vi "Read Register.vi"() -> ()   [LabVIEW 2013]
uses:
  HSDIO/MIPI_RFFE/Ctrls/Configuration.ctl
  HSDIO/MIPI_RFFE/Ctrls/ClockDataChannels.ctl
  HSDIO/MIPI_RFFE/Ctrls/RegReadWrite.ctl
  <vilib>/NI_TestStand_SemiconductorModule/NI_TestStand_Semiconductor_Module.lvlibp/PinMap/General/SemiconductorModuleContext.ctl
  <vilib>/NI_TestStand_SemiconductorModule/NI_TestStand_Semiconductor_Module.lvlibp/PinMap/HSDIO/PinsToNIHSDIOSession.vi
  <instrlib>/niHSDIO/niHSDIO.llb/niHSDIO Write Named Waveform (WDT).vi
  <instrlib>/niHSDIO/niHSDIO.llb/niHSDIO Fetch Waveform (WDT).vi
  <vilib>/NI_TestStand_SemiconductorModule/NI_TestStand_Semiconductor_Module.lvlibp
panel:
  in  "Semiconductor Module Context":T1
  in  "Pins":string[](array[string])=["CLK", "SDA", "SETID"]
  out "Converted Data":T2 {"Register" max=31 format="%.0x"; "Slave Address" max=15 format="%.0x"}
  in  "Readback Speed":enum16{"Full Speed", "Half Speed"}(ring)
  in  "Data":T3 {"Register" max=31 format="%.0x"; "Slave Address" max=15 format="%.0x"}
  in  "Configuratation":T4={"Samples to Allocate"=10000, "Oversample Factor"=1, "Clock Channel"=enum."0", "Data Channel"=enum."1"} {"Oversample Factor" min=1 max=254; "Samples to Allocate" min=1}
  out "Waveform Graph":digitalwaveform(graph)
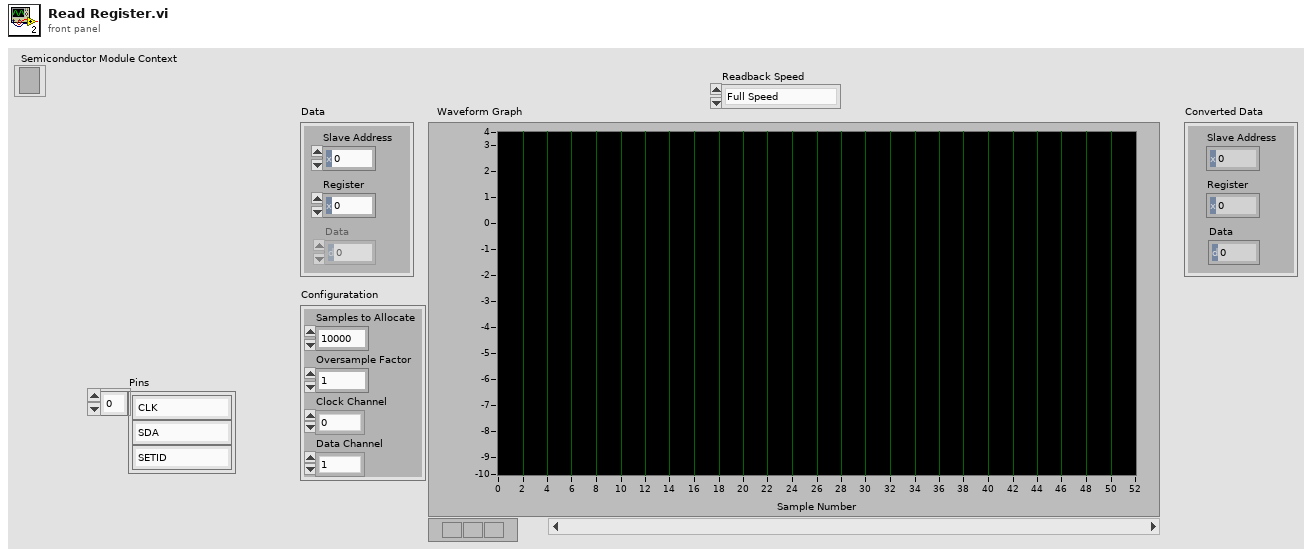
[diagram p1: front panel]
types:
  T1 = typedef "NI_TestStand_Semiconductor_Module.lvlibp/SemiconductorModuleContext.ctl" = refnum<k7>
  T2 = cluster{"Slave Address":u8, "Register":u8, "Data":u8}
  T3 = typedef "RegReadWrite.ctl" = cluster{"Slave Address":u8, "Register":u8, "Data":u8}
  T4 = typedef "Configuration.ctl" = cluster{"Samples to Allocate":i32, "Oversample Factor":u8, "Clock Channel":T5, "Data Channel":T5}
  T5 = typedef "ClockDataChannels.ctl" = enum16{"0", "1"}
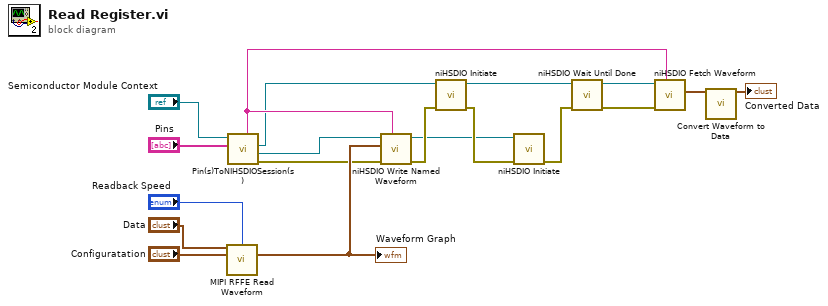
[diagram p0: block diagram]
diagram:
  n1 = call "MIPI RFFE Read Waveform.vi"("Data"="Data", "Readback Speed"="Readback Speed", "Configuratation"="Configuratation") -> ("Waveform Graph"=w14:digitalwaveform)  [unwired: 10 in, 2 out]
  "Waveform Graph" <- w14
  n2 = call-poly <vilib>:"Pin(s)ToNIHSDIOSession(s).vi"("Pins"="Pins", "Semiconductor Module Context"="Semiconductor Module Context") -> ("error out"=w5:errorcluster, "Generation Session"=w4:refnum<k15>, "Acquisition Session"=w3:refnum<k15>, "Channel List"=w17:string)  [unwired: 4 in, 2 out]
  n3 = call-poly <instrlib>:"niHSDIO Write Named Waveform.vi"("waveform name (default:\"\")"=w17, "error in (no error)"=w5, "data"=w14, "instrument handle"=w4) -> ("error out"=w6:errorcluster, "instrument handle out"=w2:refnum<k15>)  [unwired: 6 in]
  n4 = call <instrlib>:"niHSDIO Initiate.vi"("error in (no error)"=w6, "instrument handle"=w3) -> ("error out"=w12:errorcluster, "instrument handle out"=w13:refnum<k15>)  [unwired: 8 in]
  n5 = call <instrlib>:"niHSDIO Initiate.vi"("error in (no error)"=w12, "instrument handle"=w2) -> ("error out"=w11:errorcluster)  [unwired: 8 in, 1 out]
  n6 = call <instrlib>:"niHSDIO Wait Until Done.vi"("error in (no error)"=w11, "instrument handle"=w13) -> ("error out"=w10:errorcluster, "instrument handle out"=w9:refnum<k15>)  [unwired: 8 in]
  n7 = call-poly <instrlib>:"niHSDIO Fetch Waveform.vi"("channel list"=w17, "error in (no error)"=w10, "instrument handle"=w9) -> ("data"=w7:digitalwaveform)  [unwired: 5 in, 3 out]
  n8 = call "Convert Waveform to Data.vi"("Waveform Graph"=w7) -> ("Converted Data"=→"Converted Data":T2)  [unwired: 14 in]
